vi "ClsSendCmds.vi"   [LabVIEW 2015]
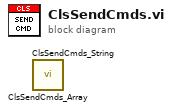
[diagram p0: block diagram]
diagram:
  n1 = call "ClsSendCmds_Array.vi"() -> ()  [unwired: 9 in, 3 out]
  n2 = call "ClsSendCmds_String.vi"() -> ()  [unwired: 9 in, 3 out]
